vi "Configuration Reference.vi"(8 "Error in":errorcluster, 11 "INL DNL Test in":refnum<class "INL DNL Test.lvclass">) -> (0 "Error out":errorcluster, 1 "Configuration Ref":refnum<vi>, 2 "VI Ref":refnum<vi>, 3 "INL DNL Test out":refnum<class "INL DNL Test.lvclass">)   [LabVIEW 2020, in "INL DNL Test.lvclass"]
uses:
  INL DNL Test.lvclass
  Configuration Page.vi
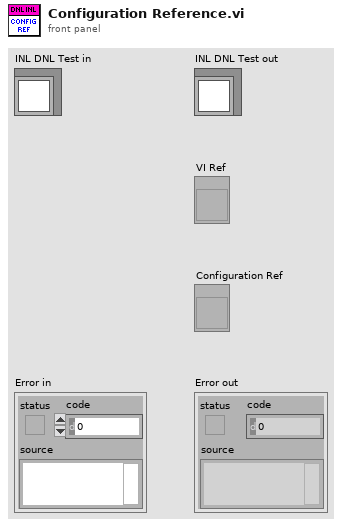
[diagram p1: front panel]
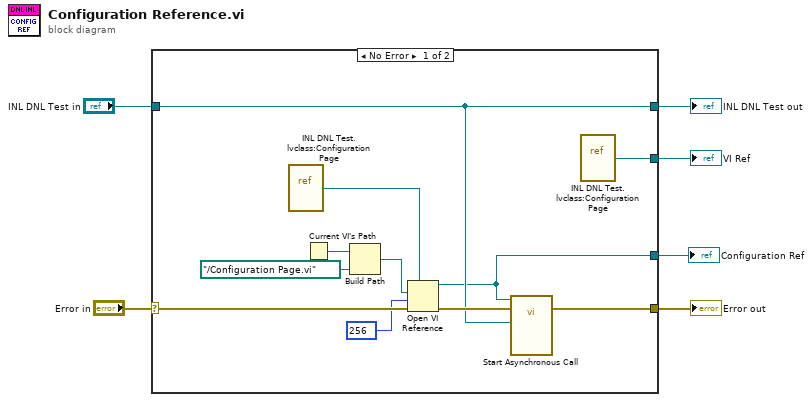
[diagram p0: block diagram]
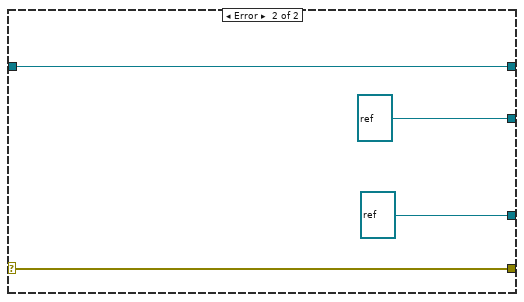
[diagram p2: hidden frame]
diagram:
  n1 = case shown="No Error" "Error in" {
    selector: "Error in" -> [w14 w21]
    tunnel: [w8 w21] -> w5
    tunnel: [w9 w20] -> w3
    tunnel: "INL DNL Test in" -> [w9 w20]
    tunnel: [w17 refnum<vi> refnum] -> w2
    tunnel: [w7 refnum<vi> refnum] -> w1
    frame No Error {
      n2 = vi-ref "INL DNL Test.lvclass:Configuration Page.vi"() -> (w12:refnum<vi>)
      n3 = Current VI's Path() -> (path=w16:path)
      n4 = Build Path(base path=w16, name or relative path=path "../Configuration Page.vi") -> (appended path=w13:path)
      n5 = Open VI Reference(type specifier VI Refnum (for type only)=w12, vi path=w13, options=256, error in (no error)=w14) -> (vi reference=w7:refnum<vi>, error out=w10:errorcluster)  [unwired: 2 in]
      n6 = call-by-ref "Start Asynchronous Call"(reference=w7, error in=w10, "INL DNL Test in"=w9) -> (error out=w8:errorcluster)  [unwired: 9 in, 3 out]
      n7 = vi-ref "INL DNL Test.lvclass:Configuration Page.vi"() -> (w17:refnum<vi>)
    }
    frame Error {
    }
  }
  "Error out" <- w5
  "INL DNL Test out" <- w3
  "VI Ref" <- w2
  "Configuration Ref" <- w1
